vi "MTM2_getEvent_authList.vi"(8 "error in (no error)":errorcluster, 11 "logevent_authList_Ctl":T1) -> (0 "error out":errorcluster, 2 "function return":i32, 3 "logevent_authList_Ctl out":T1)   [LabVIEW 2018, in "SALLV_MTM2.lvlib"]
doc: "int MTM2_shm_getEvent_authListLV(MTM2_logevent_authListLV *logevent_authList_Ctl );"
uses:
  DataTypes/logevent_authList.ctl
  SALLV_MTM2.lvlib
  SALLV_MTM2.so
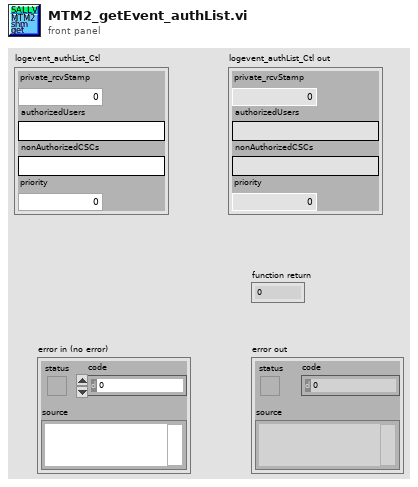
[diagram p1: front panel]
types:
  T1 = typedef "SALLV_MTM2.lvlib/logevent_authList.ctl" = cluster{"private_rcvStamp":dbl, "authorizedUsers":string, "nonAuthorizedCSCs":string, "priority":i32}
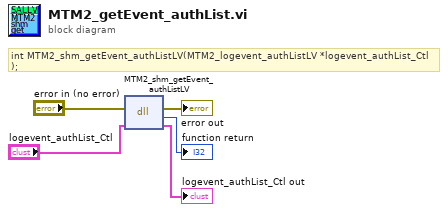
[diagram p0: block diagram]
diagram:
  # "int MTM2_shm_getEvent_authListLV(MTM2_logevent_authListLV *logevent_authList_Ctl );"
  n1 = dll-call lib="home/ttsai/Documents/salLabviewApi/SALLV_MTM2/SALLV_MTM2.*" fn="MTM2_shm_getEvent_authListLV"(error in="error in (no error)", "logevent_authList_Ctl"="logevent_authList_Ctl") -> (error out=→"error out":errorcluster, →"function return":i32, "logevent_authList_Ctl"=→"logevent_authList_Ctl out":T1)  [unwired: 2 in, 1 out]
